vi "Read Region.vi"(8 "error in (no error)":errorcluster, 11 "AWS Core in":refnum<class "AWS Core.lvclass">) -> (0 "error out":errorcluster, 2 "Region":T1, 3 "AWS Core out":refnum<class "AWS Core.lvclass">)   [LabVIEW 2015, in "NI_AWS Core.lvlib" / "AWS Core.lvclass"]
uses:
  AWS Core.lvclass
  Region.ctl
  AWS Core.lvclass/AWS Core.ctl
  NI_AWS Core.lvlib
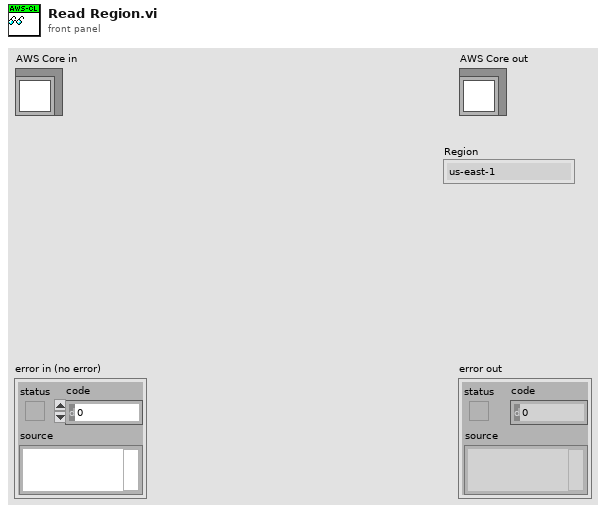
[diagram p1: front panel]
types:
  T1 = typedef "NI_AWS Core.lvlib/Region.ctl" = enum16{"us-east-1", "us-east-2", "us-west-1", "us-west-2", "ap-northeast-1", "ap-northeast-2", "ap-southeast-1", "ap-southeast-2", "ca-central-1", "eu-central-1", "eu-west-1", "eu-west-2", "sa-east-1"}
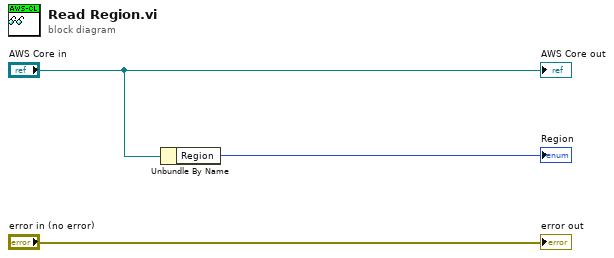
[diagram p0: block diagram]
diagram:
  n1 = Unbundle By Name("AWS Core in") -> ("Region"=→"Region":T1)
  "error out" <- "error in (no error)"
  "AWS Core out" <- "AWS Core in"
